vi "start.vi"(8 "error in (no error)":errorcluster, 11 "DistanceGauge in":refnum<class "DistanceGauge.lvclass">) -> (0 "error out":errorcluster, 3 "DistanceGauge out":refnum<class "DistanceGauge.lvclass">)   [LabVIEW 2013, in "DistanceGauge.lvclass"]
uses:
  DistanceGauge.lvclass
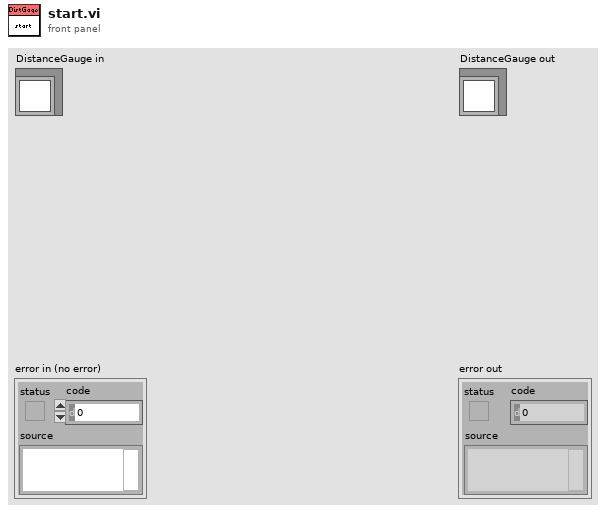
[diagram p1: front panel]
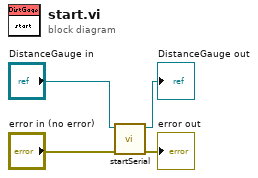
[diagram p0: block diagram]
diagram:
  n1 = call "startSerial.vi"("error in (no error)"="error in (no error)", "DistanceGauge in"="DistanceGauge in") -> ("error out"=→"error out":errorcluster, "DistanceGauge out"=→"DistanceGauge out":refnum<class "DistanceGauge.lvclass">)  [unwired: 8 in]
